vi "Init.vi"(10 "String":string) -> (3 "Hello World Msg Strategy out":refnum<class "Hello World Msg Strategy.lvclass">)   [LabVIEW 2021, in "Hello World Event.lvlib" / "Hello World Msg Strategy.lvlib" / "Hello World Msg Strategy.lvclass"]
uses:
  Hello World Msg Strategy.lvclass
  Hello World Msg Strategy.lvclass/Hello World Msg Strategy.ctl
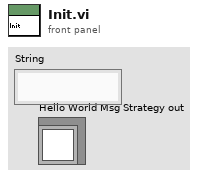
[diagram p1: front panel]
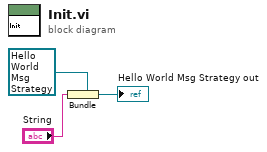
[diagram p0: block diagram]
diagram:
  n1 = Bundle "Bundle"(cluster=refnum<class "Hello World Msg Strategy.lvclass"> refnum ("TEMPLATE Msg Strategy out"), "String") -> (→"Hello World Msg Strategy out":refnum<class "Hello World Msg Strategy.lvclass">)
